vi "DeurOpdracht.vi"   [LabVIEW 2014, in "LegoMindstormProjects.lvrbt"]
uses:
  LegoMindstormProjects.lvrbt
  <vilib>/NXT/Block Support/NXT_InputPort.ctl
  <vilib>/NXT/Subs/ColorSensorColors.ctl
  <vilib>/NXT/Block Support/NXT_OutputPort.ctl
  <vilib>/NXT/Dual Mode Library/Sensors/EV3_Gyro_Reset.vi
  <vilib>/NXT/NXTIO Xnodes/NXTIONodeSubVIs/NXTMoveMotors.vi
  <vilib>/NXT/Dual Mode Library/Waits/Wait_EV3_Ultrasonic_Centimeter_Closer.vi
  <vilib>/NXT/NXTIO Xnodes/NXTIONodeSubVIs/NXTStopMotors.vi
  <vilib>/NXT/Dual Mode Library/Waits/Wait_Rotation.vi
  <vilib>/NXT/Dual Mode Library/Waits/Wait_EV3_Color_Color.vi
  <vilib>/NXT/Dual Mode Library/Waits/Wait_EV3_Angle_Greater.vi
  <vilib>/NXT/NXTIO Xnodes/AddressXNode/NXTIOAddress.xnode
  <vilib>/NXT/NXTIO Xnodes/NXTIOXNode/NXTIO.xnode
  <vilib>/NXT/Subs/LVHSConnector.ctl
  <vilib>/NXT/LegoClasses/BrickReference/BrickReference.lvclass
types:
  T1 = typedef "NXT_InputPort.ctl" = u32
  T2 = typedef "NXT_OutputPort.ctl" = u8
  T3 = typedef "ColorSensorColors.ctl" = enum16{"No Color", "Black", "Blue", "Green", "Yellow", "Red", "White", "Brown"}
  T4 = typedef "LVHSConnector.ctl" = refnum<class "BrickReference.lvclass">
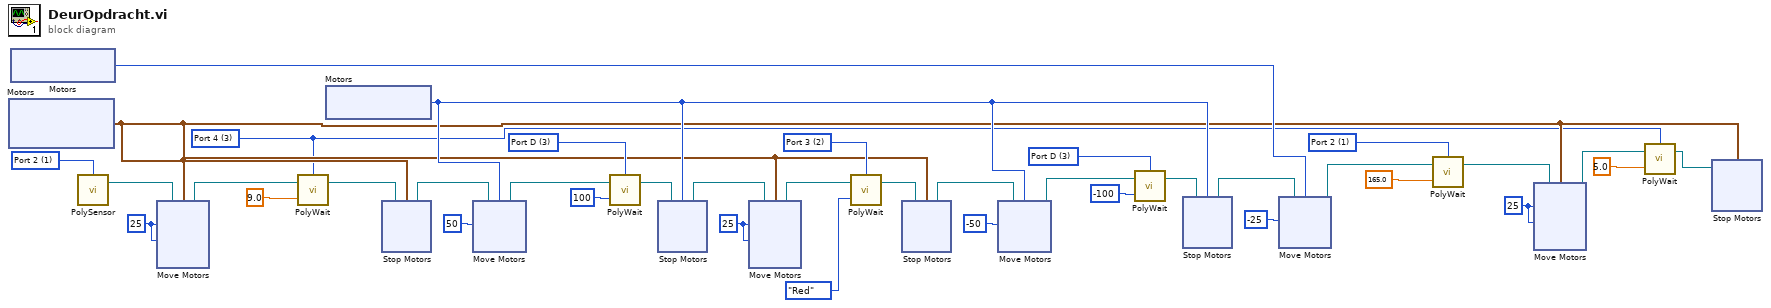
[diagram p0: block diagram]
diagram:
  w7 = i8 25 ("Power/Speed 2")
  w9 = T1 1 items=["Port 1", "Port 2", "Port 3", "Port 4"] ("Port (Port 1)")
  w13 = T1 1 items=["Port 1", "Port 2", "Port 3", "Port 4"] ("Port (Port 1)")
  w19 = T2 3 items=["Port A", "Port B", "Port C", "Port D"] ("Port (Port A)")
  w6 = T1 2 items=["Port 1", "Port 2", "Port 3", "Port 4"] ("Port (Port 1)")
  w17 = i8 25 ("Power/Speed 1")
  w30 = T2 3 items=["Port A", "Port B", "Port C", "Port D"] ("Port (Port A)")
  w1 = T1 3 items=["Port 1", "Port 2", "Port 3", "Port 4"] ("Port (Port 1)")
  w38 = i8 25 ("Power/Speed 1")
  n1 = xnode "Motors"() -> ("Motor"=w5:cluster{"Port":T2, "Port":T2})
  n2 = xnode "Motors"() -> ("Motor"=w16:T2)
  n3 = call-poly <vilib>:"PolySensor.vi"("Port (Port 1)"=w13) -> ("NXT/EV3"=w14:T4)  [unwired: 3 in]
  n4 = xnode "Move Motors"("Power/Speed 2"=w38, "Power/Speed 1"=w38, "Motors"=w5, "NXT/EV3"=w14) -> ("NXT/EV3"=w36:T4)
  n5 = call-poly <vilib>:"PolyWait.vi"("Centimeters (40)"=sgl 9.0, "NXT/EV3"=w36, "Port (Port 1)"=w1) -> ("NXT/EV3"=w35:T4)  [unwired: 1 in]
  n6 = xnode "Motors"() -> ("Motor"=w18:T2)
  n7 = xnode "Stop Motors"("Motors"=w5, "NXT/EV3"=w35) -> ("NXT/EV3"=w34:T4)
  n8 = xnode "Move Motors"("Power/Speed 1"=i8 50, "Motors"=w18, "NXT/EV3"=w34) -> ("NXT/EV3"=w32:T4)
  n9 = call-poly <vilib>:"PolyWait.vi"("Position Change (180)"=100, "NXT/EV3"=w32, "Port (Port A)"=w30) -> ("NXT/EV3"=w26:T4)  [unwired: 1 in]
  n10 = xnode "Stop Motors"("Motors"=w18, "NXT/EV3"=w26) -> ("NXT/EV3"=w25:T4)
  n11 = xnode "Move Motors"("Power/Speed 2"=w17, "Power/Speed 1"=w17, "Motors"=w5, "NXT/EV3"=w25) -> ("NXT/EV3"=w28:T4)
  n12 = call-poly <vilib>:"PolyWait.vi"("Color (Red)"=ColorSensorColors."Red", "NXT/EV3"=w28, "Port (Port 1)"=w6) -> ("NXT/EV3"=w27:T4)  [unwired: 1 in]
  n13 = xnode "Stop Motors"("Motors"=w5, "NXT/EV3"=w27) -> ("NXT/EV3"=w24:T4)
  n14 = xnode "Move Motors"("Power/Speed 1"=i8 -50, "Motors"=w18, "NXT/EV3"=w24) -> ("NXT/EV3"=w23:T4)
  n15 = call-poly <vilib>:"PolyWait.vi"("Position Change (180)"=-100, "NXT/EV3"=w23, "Port (Port A)"=w19) -> ("NXT/EV3"=w22:T4)  [unwired: 1 in]
  n16 = xnode "Stop Motors"("Motors"=w18, "NXT/EV3"=w22) -> ("NXT/EV3"=w12:T4)
  n17 = xnode "Move Motors"("Power/Speed 1"=i8 -25, "Motors"=w16, "NXT/EV3"=w12) -> ("NXT/EV3"=w10:T4)
  n18 = call-poly <vilib>:"PolyWait.vi"("Degrees (180)"=sgl 165.0, "NXT/EV3"=w10, "Port (Port 1)"=w9) -> ("NXT/EV3"=w8:T4)  [unwired: 1 in]
  n19 = xnode "Move Motors"("Power/Speed 2"=w7, "Power/Speed 1"=w7, "Motors"=w5, "NXT/EV3"=w8) -> ("NXT/EV3"=w2:T4)
  n20 = call-poly <vilib>:"PolyWait.vi"("Centimeters (40)"=sgl 5.0, "NXT/EV3"=w2, "Port (Port 1)"=w1) -> ("NXT/EV3"=w3:T4)  [unwired: 1 in]
  n21 = xnode "Stop Motors"("Motors"=w5, "NXT/EV3"=w3) -> ()  [unwired: 1 out]
